vi "LEDs Shift Step.vi"(11 "Interpolate Out":T1(array[cluster])) -> (0 "Done":bool, 2 "LED Bit Array":u8[](array[numeric]), 3 "Array":T1(array[cluster]))   [LabVIEW 2014]
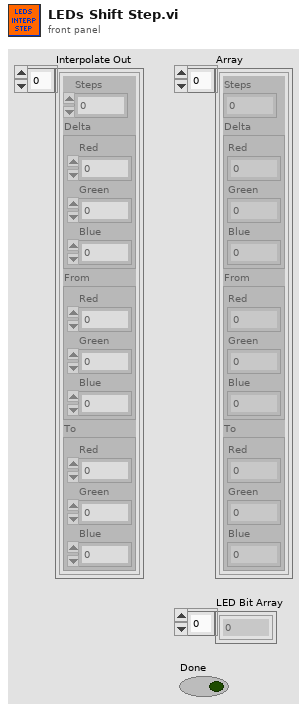
[diagram p1: front panel]
types:
  T1 = cluster{"Steps":i32, "Delta":cluster{"Red":dbl, "Green":dbl, "Blue":dbl}, "From":cluster{"Red":dbl, "Green":dbl, "Blue":dbl}, "To":cluster{"Red":dbl, "Green":dbl, "Blue":dbl}}[]
  T2 = cluster{"Steps":i32, "Delta":cluster{"Red":dbl, "Green":dbl, "Blue":dbl}, "From":cluster{"Red":dbl, "Green":dbl, "Blue":dbl}, "To":cluster{"Red":dbl, "Green":dbl, "Blue":dbl}}
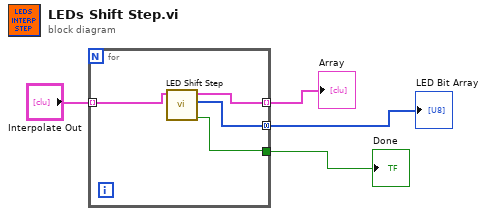
[diagram p0: block diagram]
diagram:
  n1 = for {
    tunnel: "Interpolate Out" -> [w8] mode=indexing
    tunnel: [w7] -> w3 mode=indexing
    tunnel: [w6] -> w2 mode=concatenating
    tunnel: [w5] -> w4
    n2 = call "LED Shift Step.vi"("LED Interpolate In"=w8) -> ("Done"=w5:bool, "LED Bit Array"=w6:u8[], "LED Interpolate Out"=w7:T2)  [unwired: 7 in]
  }
  "Done" <- w4
  "Array" <- w3
  "LED Bit Array" <- w2
